vi "Quit.vi"(8 "error in (no error)":errorcluster, 11 "Log Sinks in":refnum<class "Log Sinks.lvclass">) -> (0 "error out":errorcluster, 3 "Log Sinks final":refnum<class "Log Sinks.lvclass">)   [LabVIEW 2019, in "TSC Event Logger.lvlib" / "Log Sinks.lvclass"]
doc: "Close the queue reference of the log sink.\n\n<b>Code Developed By:</b>\nTechnology Service Corporation\nBloomington, IN 47403\nwww.tsc.com/atcs\n\nDeveloper:\nDaniel Coons"
uses:
  Log Sinks.lvclass
  Log Sinks.lvclass/Log Sinks.ctl
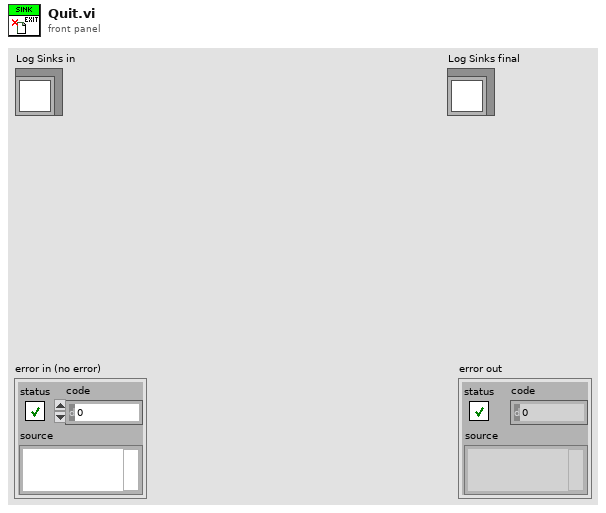
[diagram p1: front panel]
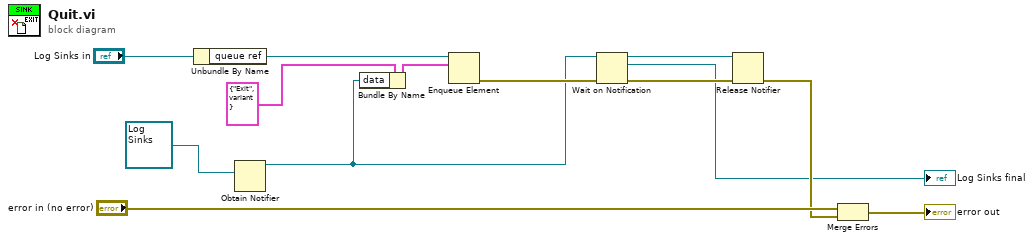
[diagram p0: block diagram]
diagram:
  n1 = Unbundle By Name("Log Sinks in") -> ("queue ref"=w11:refnum<queue>)
  n2 = Obtain Notifier(notification data type=refnum<class "Log Sinks.lvclass"> refnum ("Log Sinks final")) -> (notifier out=w1:refnum<notifier>)  [unwired: 3 in, 2 out]
  n3 = Bundle By Name(cluster=cluster{"msg":string, "data":variant} {"msg"="Exit", "data"=variant} ("element"), "data"=w1) -> (w2:cluster{"msg":string, "data":variant})
  n4 = Enqueue Element(queue=w11, element=w2) -> (error out=w8:errorcluster)  [unwired: 2 in, 2 out]
  n5 = Wait on Notification(notifier=w1, error in (no error)=w8) -> (notifier out=w4:refnum<notifier>, notification=→"Log Sinks final":refnum<class "Log Sinks.lvclass">, error out=w6:errorcluster)  [unwired: 2 in, 1 out]
  n6 = Release Notifier(notifier=w4, error in (no error)=w6) -> (error out=w5:errorcluster)  [unwired: 1 in, 2 out]
  n7 = Merge Errors("error in (no error)", w5) -> (→"error out":errorcluster)
